vi "Complete Call.vi"(0 "gRPCid":T1, 3 "error in (no error)":errorcluster) -> (10 "error out":errorcluster)   [LabVIEW 2019, in "TestServer.lvlib" / "gprc-lvsupport.lvlib"]
uses:
  gprc-lvsupport.lvlib
  typeDefs/grpcId.ctl
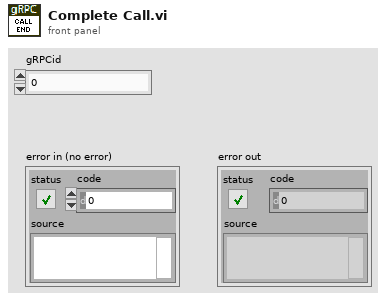
[diagram p1: front panel]
types:
  T1 = typedef "TestServer.lvlib/gprc-lvsupport.lvlib/grpcId.ctl" = u64
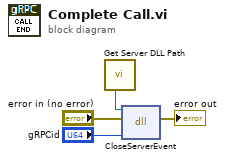
[diagram p0: block diagram]
diagram:
  n1 = call "Get Server DLL Path.vi"() -> ("Server dll path"=w1:path)
  n2 = dll-call lib="C:/Users/XEnderMD/Desktop/LV gRPC/labview source/gRPC interface/dlls/labview_grpc_server.dll" fn="CloseServerEvent"(path in=w1, error in="error in (no error)", "id"="gRPCid") -> (error out=→"error out":errorcluster)  [unwired: 3 in, 1 out]
